vi "Range_set (SubVI).vi"(9 "RangeChB":T1(ring), 10 "RangeChA":T1(ring), 11 "A5000_param in":T2 {"Arbitrary Waveform Settings"."Index Mode" items=["Single", "Dual", "Quad"]; "Standard Waveform Settings"."Stop Frequency" min=0.03 max=1000000.0; "Standard Waveform Settings"."Start Frequency" min=0.03 max=1000000.0; "General AWG Settings"."White Noise/PRBS" items=["Normal", "White Noise", "PRBS"]; "General AWG Settings"."Trigger Source" items=["None", "Scope Trigger", "Aux. In", "Ext. In", "Software Trigger"]; "General AWG Settings"."Trigger Type" items=["Rising", "Falling", "Gate High", "Gate Low"]; "General AWG Settings"."Sweep Type" items=["Up", "Down", "Up-Down", "Down-Up"]; "General AWG Settings"."Wave Type" items=["Sine", "Square", "Triangle", "Ramp Up", "Ramp Down", "Sinc", "Gaussian", "Half Sine", "DC", "Arbitrary"]; "Resolution" items=["8-bit", "12-bit", "14-bit", "15-bit (max. 2 ch.)", "16-bit (max. 1 ch.)"]; "Properties"."Max Total Capture Time Available (sec)" format="%.3p"; "Properties"."Sample Frequency" format="%.3p"; "Properties"."Sample Rate" format="%.3p"; "Properties"."Max Samples Available" format="%.3p"; "Properties"."Total Capture Time (sec)" format="%.3p"; "Acquisition"."Down Sample Ratio" min=1 step=1; "Acquisition"."Down-Sample Mode" items=["None"=0, "Aggregate"=1, "Decimate"=2, "Average"=4]; "Trigger"."Trigger Direction" items=["Rising"=2, "Falling"=3]; "ChannelB"."Range" items=["10 mV", "20 mV", "50 mV", "100 mV", "200 mV", "500 mV", "1 V", "2 V", "5 V", "10 V", "20 V"]; "ChannelB"."Coupling" items=["AC", "DC"]; "ChannelA"."Range" items=["10 mV", "20 mV", "50 mV", "100 mV", "200 mV", "500 mV", "1 V", "2 V", "5 V", "10 V", "20 V"]; "ChannelA"."Coupling" items=["AC", "DC"]}) -> (3 "A5000_param out 2":T2 {"Arbitrary Waveform Settings"."Index Mode" items=["Single", "Dual", "Quad"]; "Standard Waveform Settings"."Stop Frequency" min=0.03 max=1000000.0; "Standard Waveform Settings"."Start Frequency" min=0.03 max=1000000.0; "General AWG Settings"."White Noise/PRBS" items=["Normal", "White Noise", "PRBS"]; "General AWG Settings"."Trigger Source" items=["None", "Scope Trigger", "Aux. In", "Ext. In", "Software Trigger"]; "General AWG Settings"."Trigger Type" items=["Rising", "Falling", "Gate High", "Gate Low"]; "General AWG Settings"."Sweep Type" items=["Up", "Down", "Up-Down", "Down-Up"]; "General AWG Settings"."Wave Type" items=["Sine", "Square", "Triangle", "Ramp Up", "Ramp Down", "Sinc", "Gaussian", "Half Sine", "DC", "Arbitrary"]; "Resolution" items=["8-bit", "12-bit", "14-bit", "15-bit (max. 2 ch.)", "16-bit (max. 1 ch.)"]; "Properties"."Max Total Capture Time Available (sec)" format="%.3p"; "Properties"."Sample Frequency" format="%.3p"; "Properties"."Sample Rate" format="%.3p"; "Properties"."Max Samples Available" format="%.3p"; "Properties"."Total Capture Time (sec)" format="%.3p"; "Acquisition"."Down Sample Ratio" min=1 step=1; "Acquisition"."Down-Sample Mode" items=["None"=0, "Aggregate"=1, "Decimate"=2, "Average"=4]; "Trigger"."Trigger Direction" items=["Rising"=2, "Falling"=3]; "ChannelB"."Range" items=["10 mV", "20 mV", "50 mV", "100 mV", "200 mV", "500 mV", "1 V", "2 V", "5 V", "10 V", "20 V"]; "ChannelB"."Coupling" items=["AC", "DC"]; "ChannelA"."Range" items=["10 mV", "20 mV", "50 mV", "100 mV", "200 mV", "500 mV", "1 V", "2 V", "5 V", "10 V", "20 V"]; "ChannelA"."Coupling" items=["AC", "DC"]})   [LabVIEW 2017]
uses:
  controls/A5000_param.ctl
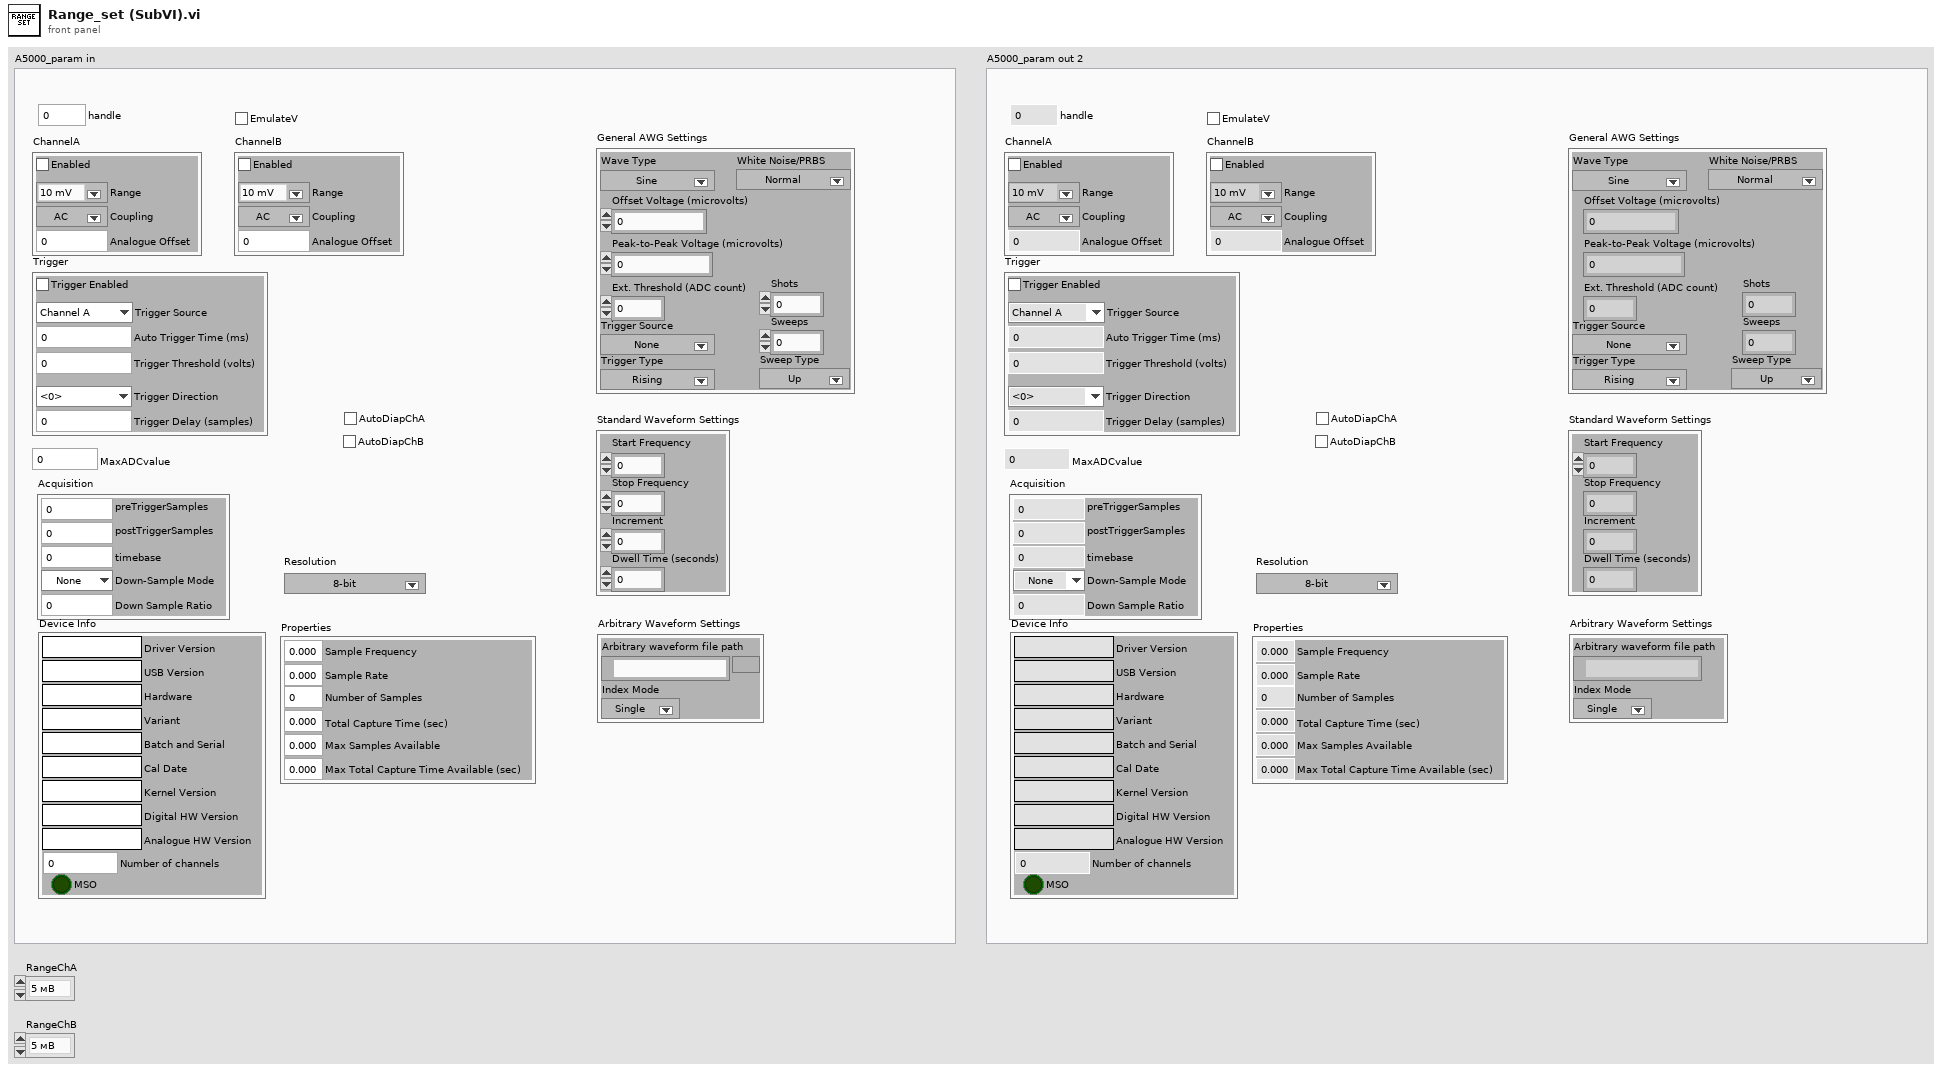
[diagram p1: front panel]
types:
  T1 = enum16{"5 мВ", "10 мВ", "25 мВ", "50 мВ", "100 мВ", "250 мВ", "0,5 В", "1,0 В", "2,5 В", "5 В", "10 В", "Авто", "Выкл."}
  T2 = typedef "A5000_param.ctl" = cluster{"ChannelA":cluster{"Enabled":bool, "Coupling":i16, "Range":u16, "Analogue Offset":sgl}, "ChannelB":cluster{"Enabled":bool, "Coupling":i16, "Range":u16, "Analogue Offset":sgl}, "Trigger":cluster{"Trigger Enabled":bool, "Trigger Source":enum16{"Channel A", "Channel B", "Channel C", "Channel D", "Ext."}, "Trigger Threshold (volts)":dbl, "Trigger Direction":u16, "Trigger Delay (samples)":u32, "Auto Trigger Time (ms)":i16}, "MaxADCvalue":i16, "handle":i16, "Acquisition":cluster{"preTriggerSamples":i32, "postTriggerSamples":i32, "timebase":u32, "Down-Sample Mode":u32, "Down Sample Ratio":u32}, "Device Info":cluster{"Driver Version":string, "USB Version":string, "Hardware":string, "Variant":string, "Batch and Serial":string, "Cal Date":string, "Kernel Version":string, "Digital HW Version":string, "Analogue HW Version":string, "MSO":bool, "Number of channels":i16}, "Properties":cluster{"Sample Frequency":sgl, "Sample Rate":sgl, "Max Samples Available":i32, "Number of Samples":u32, "Total Capture Time (sec) ":sgl, "Max Total Capture Time Available (sec)":sgl}, "Resolution":i32, "EmulateV":bool, "General AWG Settings":cluster{"Peak-to-Peak Voltage (microvolts)":u32, "Offset Voltage (microvolts)":i32, "Wave Type":u32, "Sweep Type":u32, "Shots":u32, "Sweeps":u32, "Trigger Type":u32, "Trigger Source":u32, "Ext. Threshold (ADC count)":i16, "White Noise/PRBS":u32}, "Standard Waveform Settings":cluster{"Start Frequency":dbl, "Stop Frequency":dbl, "Increment":dbl, "Dwell Time (seconds)":dbl}, "Arbitrary Waveform Settings":cluster{"Arbirary waveform file path":path, "Index Mode":u32}, "AutoDiapChA":bool, "AutoDiapChB":bool}
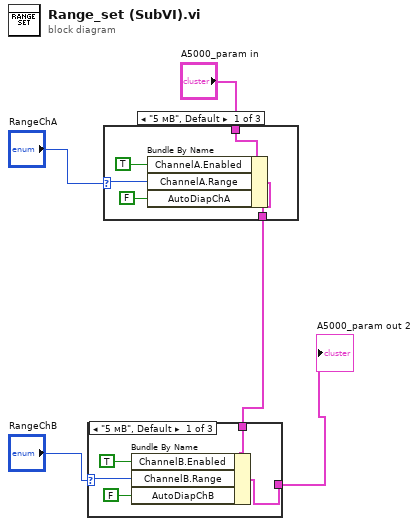
[diagram p0: block diagram]
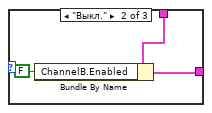
[diagram p2: hidden frame]
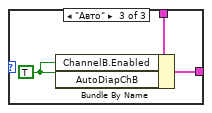
[diagram p3: hidden frame]
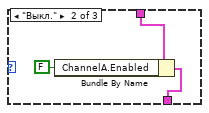
[diagram p4: hidden frame]
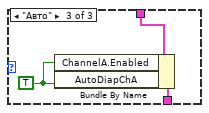
[diagram p5: hidden frame]
diagram:
  n1 = case shown="\"5 мВ\", Default" "RangeChA" {
    selector: "RangeChA" -> [w10 _ _]
    tunnel: "A5000_param in" -> [w9 w12 w16]
    tunnel: [w8 w11 w15] -> w3
    frame "5 мВ", Default {
      n2 = Bundle By Name(cluster=w9, "ChannelA.Enabled"=TRUE, "ChannelA.Range"=w10, "AutoDiapChA"=FALSE) -> (w8:T2)
    }
    frame "Выкл." {
      n3 = Bundle By Name(cluster=w12, "ChannelA.Enabled"=FALSE) -> (w11:T2)
    }
    frame "Авто" {
      w14 = TRUE ("AutoDiapChA")
      n4 = Bundle By Name(cluster=w16, "ChannelA.Enabled"=w14, "AutoDiapChA"=w14) -> (w15:T2)
    }
  }
  n5 = case shown="\"5 мВ\", Default" "RangeChB" {
    selector: "RangeChB" -> [w21 _ _]
    tunnel: w3 -> [w20 w24 w27]
    tunnel: [w19 w23 w26] -> w4
    frame "5 мВ", Default {
      n6 = Bundle By Name(cluster=w20, "ChannelB.Enabled"=TRUE, "ChannelB.Range"=w21, "AutoDiapChB"=FALSE ("AutoDiapChA")) -> (w19:T2)
    }
    frame "Выкл." {
      n7 = Bundle By Name(cluster=w24, "ChannelB.Enabled"=FALSE ("ChannelA.Enabled")) -> (w23:T2)
    }
    frame "Авто" {
      w25 = TRUE ("AutoDiapChA")
      n8 = Bundle By Name(cluster=w27, "ChannelB.Enabled"=w25, "AutoDiapChB"=w25) -> (w26:T2)
    }
  }
  "A5000_param out 2" <- w4
